vi "CalculateAngleStagetoStave.vi"(0 "Coordinates from images":dbl[][](array[numeric])=[[-618.0000019526123, 132.09984513301268, 23.216226053071207], [-618.0000015711425, 132.10001145381347, 23.216226053071207], [-618.0000001215576, 132.1000061132373, 23.216226053071207], [-606.0002838354981, 132.10000000972167, 23.216226053071207], [-605.9999977332031, 132.10000084895506, 23.216226053071207], [-605.9999913245117, 132.10000268000977, 23.216226053071207], [-337.9510112720312, 132.10002915400878, 23.21612605307121], [-337.9500060230078, 132.10001061458007, 23.216226053071207], [-337.95000091131345, 132.1000039007129, 23.216226053071207], [-325.94987751994137, 132.10000496882813, 23.216226053071207], [-325.9500149253368, 132.10000496882813, 23.216226053071207], [-325.9500006583691, 132.10000573176757, 23.216226053071207], [-43.949846358593746, 132.09996766108887, 23.216226053071207], [-43.950016265209946, 132.09999520320312, 23.216226053071207], [-43.94999185114746, 132.10000382441893, 23.216226053071207], [-31.950448924521478, 132.10000634211914, 23.21612605307121], [-31.94999062679199, 132.10001427668945, 23.216226053071207], [-31.95000397823242, 132.10000313777343, 23.216226053071207], [250.04977136382323, 132.10009530085938, 23.216226053071207], [250.04998895415525, 132.09999756831542, 23.216226053071207], [250.04999795684077, 132.10000405330078, 23.216226053071207], [262.0491744629883, 132.1000239660205, 23.21612605307121], [262.04998653574216, 132.10000451106444, 23.216226053071207], [262.05000721140135, 132.1000140478076, 23.216226053071207]], 1 "Templates path":path=path "C:/Users/Aerotech/Documents/BNL_ThermomechanicalStave/0_Calibration", 2 "Image Array":T1[](array[typedef])=["image_000_-618_132_23", "image_001_-618_132_23", "image_002_-618_132_23", "image_003_-606_132_23", "image_004_-606_132_23", "image_005_-606_132_23", "image_006_-338_132_23", "image_007_-338_132_23", "image_008_-338_132_23", "image_009_-326_132_23", "image_010_-326_132_23", "image_011_-326_132_23", "image_012_-44_132_23", "image_013_-44_132_23", "image_014_-44_132_23", "image_015_-32_132_23", "image_016_-32_132_23", "image_017_-32_132_23", "image_018_250_132_23", "image_019_250_132_23", "image_020_250_132_23", "image_021_262_132_23", "image_022_262_132_23", "image_023_262_132_23"], 3 "Pixel resolution":dbl=1.529578681813674 format="%#_13g", 5 "Number of images each":i32=3, 7 "Number of pins":i32=4) -> (4 "Angle":dbl=0.0006856978788182783, 6 "Locations pins":dbl[][](array[numeric])=[[-609.3870429531735, -329.18563865969537, -35.10730846902823, 259.01426916444484], [134.0388179973662, 135.08170067352683, 134.8703908188264, 134.78325815098862]], 8 "Each point on located edges":T3(graph)=[{"Top averages"=[-601.3926714238871, -617.3814144824598, nan, -323.4827145583182, -334.88856276107254, nan, -29.406789160441058, -40.80782777761541, nan, 264.732596858135, 253.29594147075468, nan, -609.3870429531735, -609.3870429531735, -609.3870429531735, -329.18563865969537, -329.18563865969537, -329.18563865969537, -35.10730846902823, -35.10730846902823, -35.10730846902823, 259.01426916444484, 259.01426916444484, 259.01426916444484], "Best Linear Fit"=[134.0388179973662, 134.0388179973662, 134.0388179973662, 135.08170067352683, 135.08170067352683, 135.08170067352683, 134.8703908188264, 134.8703908188264, 134.8703908188264, 134.78325815098862, 134.78325815098862, 134.78325815098862, 134.09820366135074, 133.97943233338168, nan, 135.73823170843656, 134.4251696386171, nan, 135.57292450870293, 134.16785712894986, nan, 135.40219923996895, 134.16431706200828, nan]}, {"Top averages"=[-700.0, -300.0, 100.0, 500.0, 700.0], "Best Linear Fit"=[134.3360645312021, 134.61034372571643, 134.88462292023075, 135.15890211474508, 135.29604171200225]}])   [LabVIEW 2016]
uses:
  <vilib>/Analysis/6fits.llb/Curve Fitting Criteria.ctl
  <vilib>/vision/Image Controls.llb/IMAQ Image.ctl
  <vilib>/Analysis/NI_AALPro.lvlib
panel:
  in  "Testing?":bool=TRUE
  out "Point for each edge- units":dbl[][][](array[numeric])=[[[-616.6853013924161, 133.98498133920288, 23.19072534]], [[-602.0918631529712, 134.0873275784507, 23.19072534]], [[-616.6844686564219, 133.98510562595666, 23.19072534]], [[-602.0873483929206, 134.10375101417594, 23.19072534]], [[-616.6848465163853, 133.9845728817171, 23.19072534]], [[-602.0884296079262, 134.087169544694, 23.19072534]], [[-334.3899800940794, 135.67998739590436, 23.19072534]], [[-323.9779865268114, 134.48344180918818, 23.19072534]], [[-334.3927140881534, 135.68204709551367, 23.19072534]], [[-323.98295164227596, 134.48329915078338, 23.19072534]], [[-334.3923216504359, 135.6810484407434, 23.19072534]], [[-323.97787795641597, 134.480380149028, 23.19072534]], [[-40.3112304344497, 135.51048660072627, 23.19072534]], [[-29.903300498442807, 134.22953193062764, 23.19082534]], [[-40.31259391421408, 135.5137627222535, 23.19072534]], [[-29.90268539871824, 134.2294673759651, 23.19072534]], [[-40.309615844169045, 135.51088795666246, 23.19072534]], [[-29.90442472417554, 134.2282083267235, 23.19072534]], [[253.79560124818477, 135.34840869395944, 23.19082534]], [[264.2326481830148, 134.22077460141287, 23.19082534]], [[253.79296388701863, 135.34828494250544, 23.19072534]], [[264.2354027367716, 134.217503625029, 23.19072534]], [[253.79395739751806, 135.34811629532663, 23.19072534]], [[264.23504153416127, 134.2164607476983, 23.19072534]]]
  in  "Coordinate file for image capture":path=path "C:/Users/Aerotech/cernbox/BNL/Stave Assembly Records/2017-04-07/staveCalib/staveCoordinatesSystemCaptured.csv"
  out "Filenames Array":string[](array[string])=["image_000_-618_132_23.png", "image_001_-618_132_23.png", "image_002_-618_132_23.png", "image_003_-606_132_23.png", "image_004_-606_132_23.png", "image_005_-606_132_23.png", "image_006_-338_132_23.png", "image_007_-338_132_23.png", "image_008_-338_132_23.png", "image_009_-326_132_23.png", "image_010_-326_132_23.png", "image_011_-326_132_23.png", "image_012_-44_132_23.png", "image_013_-44_132_23.png", "image_014_-44_132_23.png", "image_015_-32_132_23.png", "image_016_-32_132_23.png", "image_017_-32_132_23.png", "image_018_250_132_23.png", "image_019_250_132_23.png", "image_020_250_132_23.png", "image_021_262_132_23.png", "image_022_262_132_23.png", "image_023_262_132_23.png"]
  in  "Naming Convention":string="*.png"
  in  "Images Directory":path=path "C:/Users/Aerotech/cernbox/BNL/Stave Assembly Records/2017-04-07/staveCalib"
  out "y errors (mm)":dbl[](array[numeric])=[0.05938566398452695, 0.6565310349097196, 0.7025336898765229, 0.618941088980328]
  out "x errors (mm)":dbl[](array[numeric])=[7.994371529286357, 5.702924101377151, 5.700519308587177, 5.718327693690156]
  out "Residue":dbl=0.10525358201266499
  in  "x values for fit line on plot":dbl[](array[numeric])=[-700.0, -300.0, 100.0, 500.0, 700.0]
  out "Intercept":dbl=134.81605312160218
  in  "method":T2 items=["Least Square", "Least Absolute Residual", "Bisquare"]
  out "Slope":dbl=0.0006856979862858028
  out "Coordinate array for image capture":dbl[][](array[numeric])=[[-618.000367587, 132.100003781, 23.19072534], [-617.999992679, 132.100009503, 23.19072534], [-617.999994586, 132.100002178, 23.19072534], [-606.000466212, 132.10001202, 23.19072534], [-606.000010661, 132.100002941, 23.19072534], [-606.000002574, 132.100001492, 23.19072534], [-337.950002777, 132.100039486, 23.19072534], [-337.949993164, 132.100003857, 23.19072534], [-337.950002166, 132.099999279, 23.19072534], [-325.950148016, 132.100036511, 23.19072534], [-325.950009619, 132.100006069, 23.19072534], [-325.94999314, 132.099999279, 23.19072534], [-43.950092517, 132.099999279, 23.19072534], [-43.950004092, 132.099999279, 23.19072534], [-43.949995929, 132.100005917, 23.19072534], [-31.949232604, 132.09996014, 23.19082534], [-31.949993789, 132.100005001, 23.19072534], [-31.949996841, 132.100002178, 23.19072534], [250.05059477, 132.10003468, 23.19082534], [250.050008299, 132.099999432, 23.19072534], [250.050006239, 132.100006298, 23.19072534], [262.050305181, 132.100005917, 23.19082534], [262.050004125, 132.099996685, 23.19072534], [262.050004965, 132.100004086, 23.19072534]]
  out "Images Array":T1[](array[plugin-control])=["image_000_-618_132_23", "image_001_-618_132_23", "image_002_-618_132_23", "image_003_-606_132_23", "image_004_-606_132_23", "image_005_-606_132_23", "image_006_-338_132_23", "image_007_-338_132_23", "image_008_-338_132_23", "image_009_-326_132_23", "image_010_-326_132_23", "image_011_-326_132_23", "image_012_-44_132_23", "image_013_-44_132_23", "image_014_-44_132_23", "image_015_-32_132_23", "image_016_-32_132_23", "image_017_-32_132_23", "image_018_250_132_23", "image_019_250_132_23", "image_020_250_132_23", "image_021_262_132_23", "image_022_262_132_23", "image_023_262_132_23"]
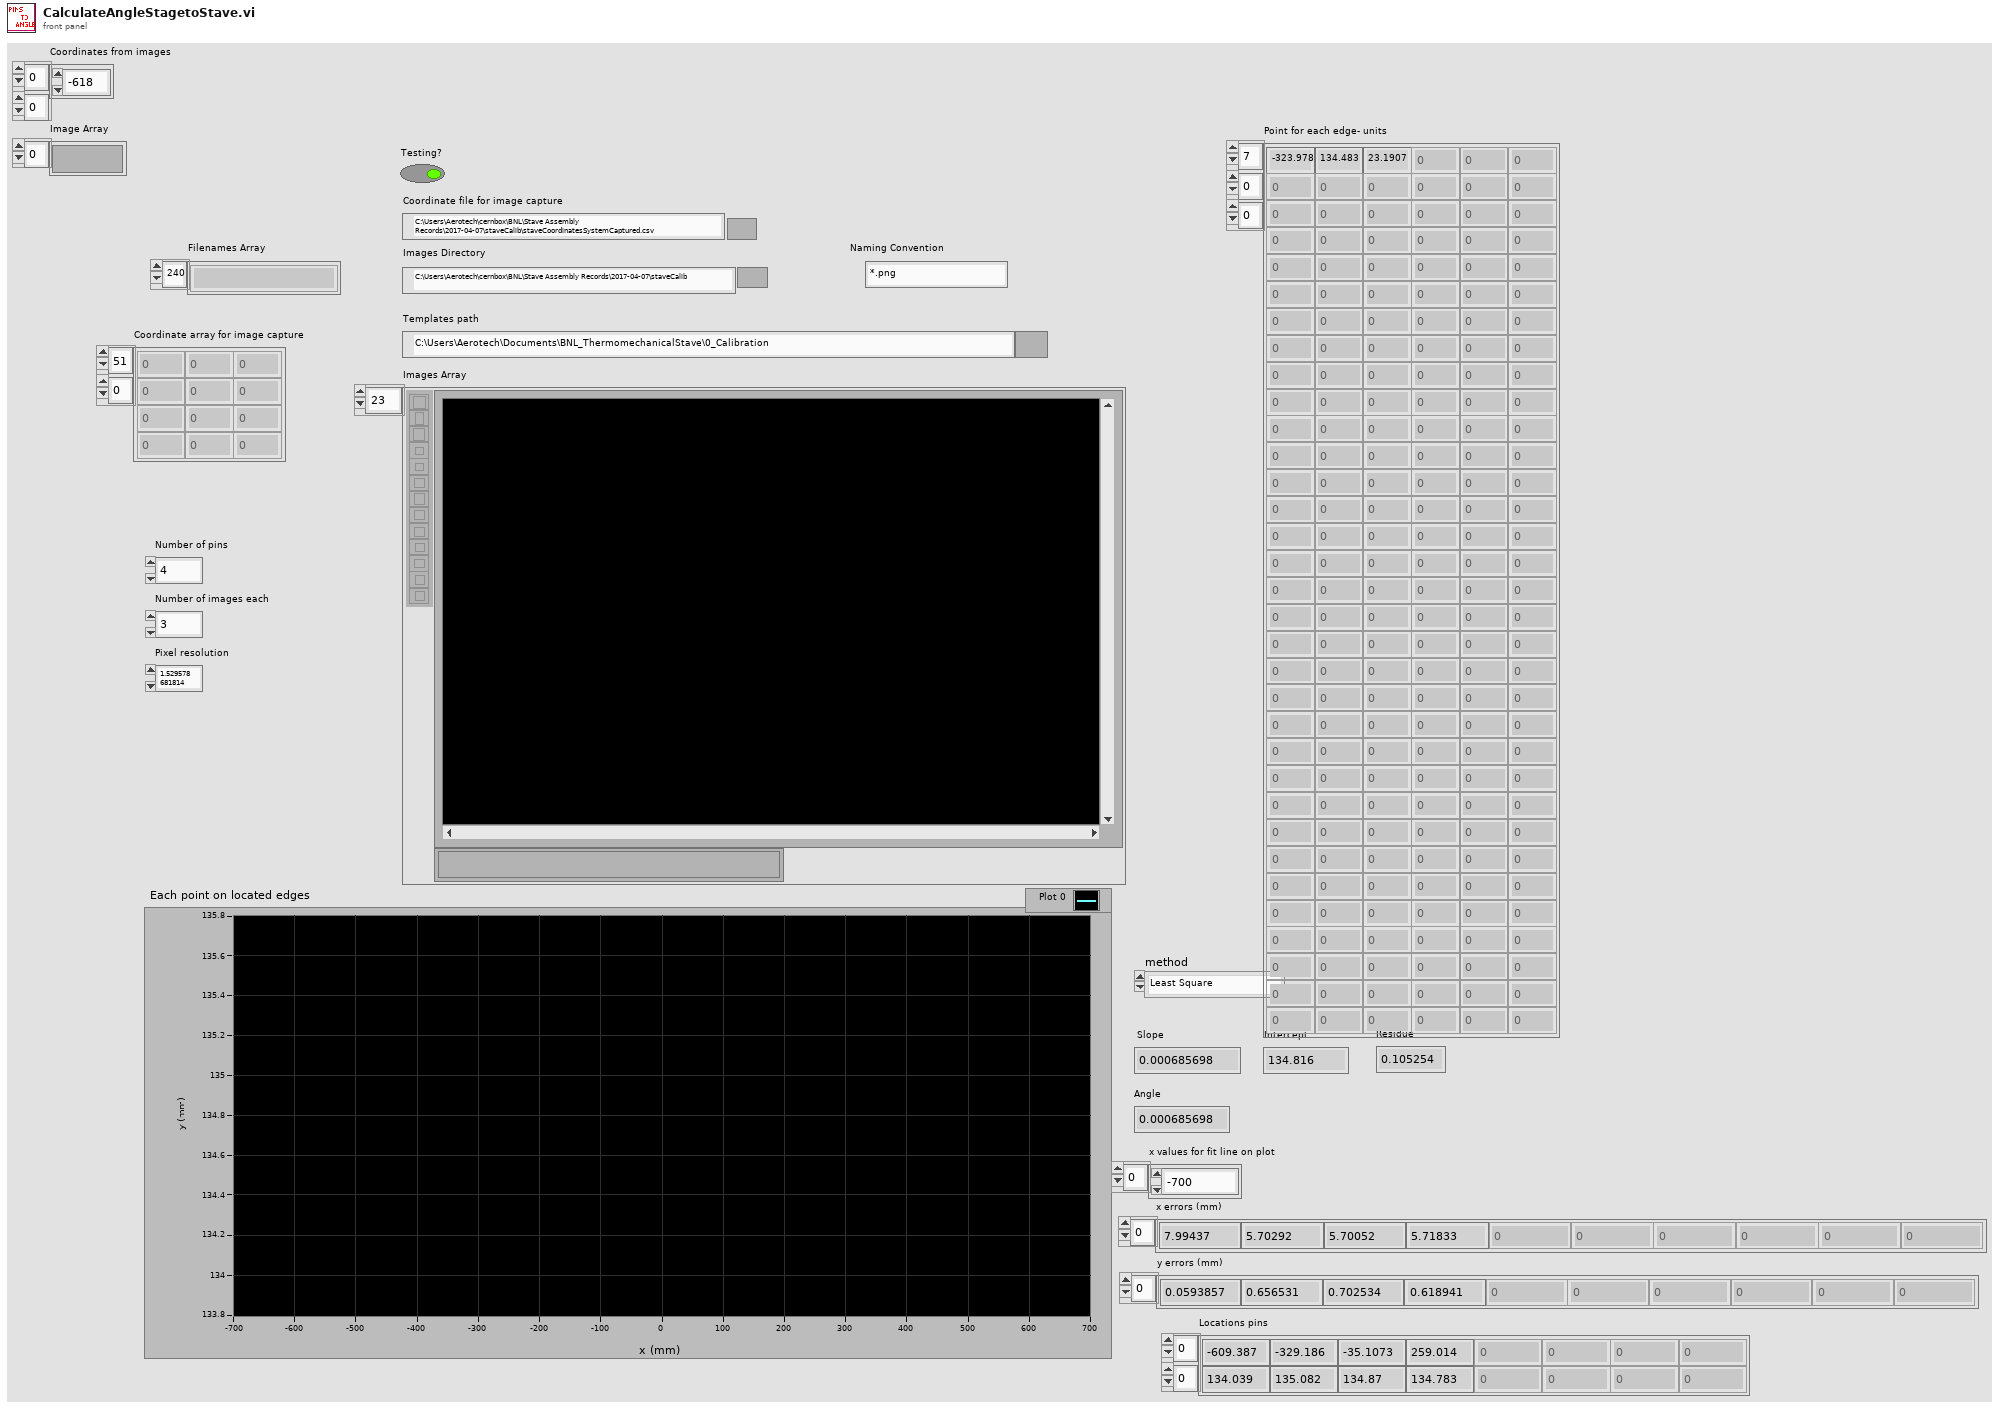
[diagram p1: front panel]
types:
  T1 = typedef "IMAQ Image.ctl" = refnum<image>
  T2 = typedef "NI_AALPro.lvlib/Curve Fitting Criteria.ctl" = u16
  T3 = cluster{"Top averages":dbl[], "Best Linear Fit":dbl[]}[]
  T4 = enum16{"cm", "mm", "pixels [mm/pix]", "pixels [um/pix]"}
  T5 = cluster{"Top Averages":dbl[], "Top Averages":dbl[]}
  T6 = cluster{"x values for fit line on plot":dbl[], "Array":dbl[]}
  T7 = cluster{"x values for fit line on plot":dbl[], "Array":dbl[]}[]
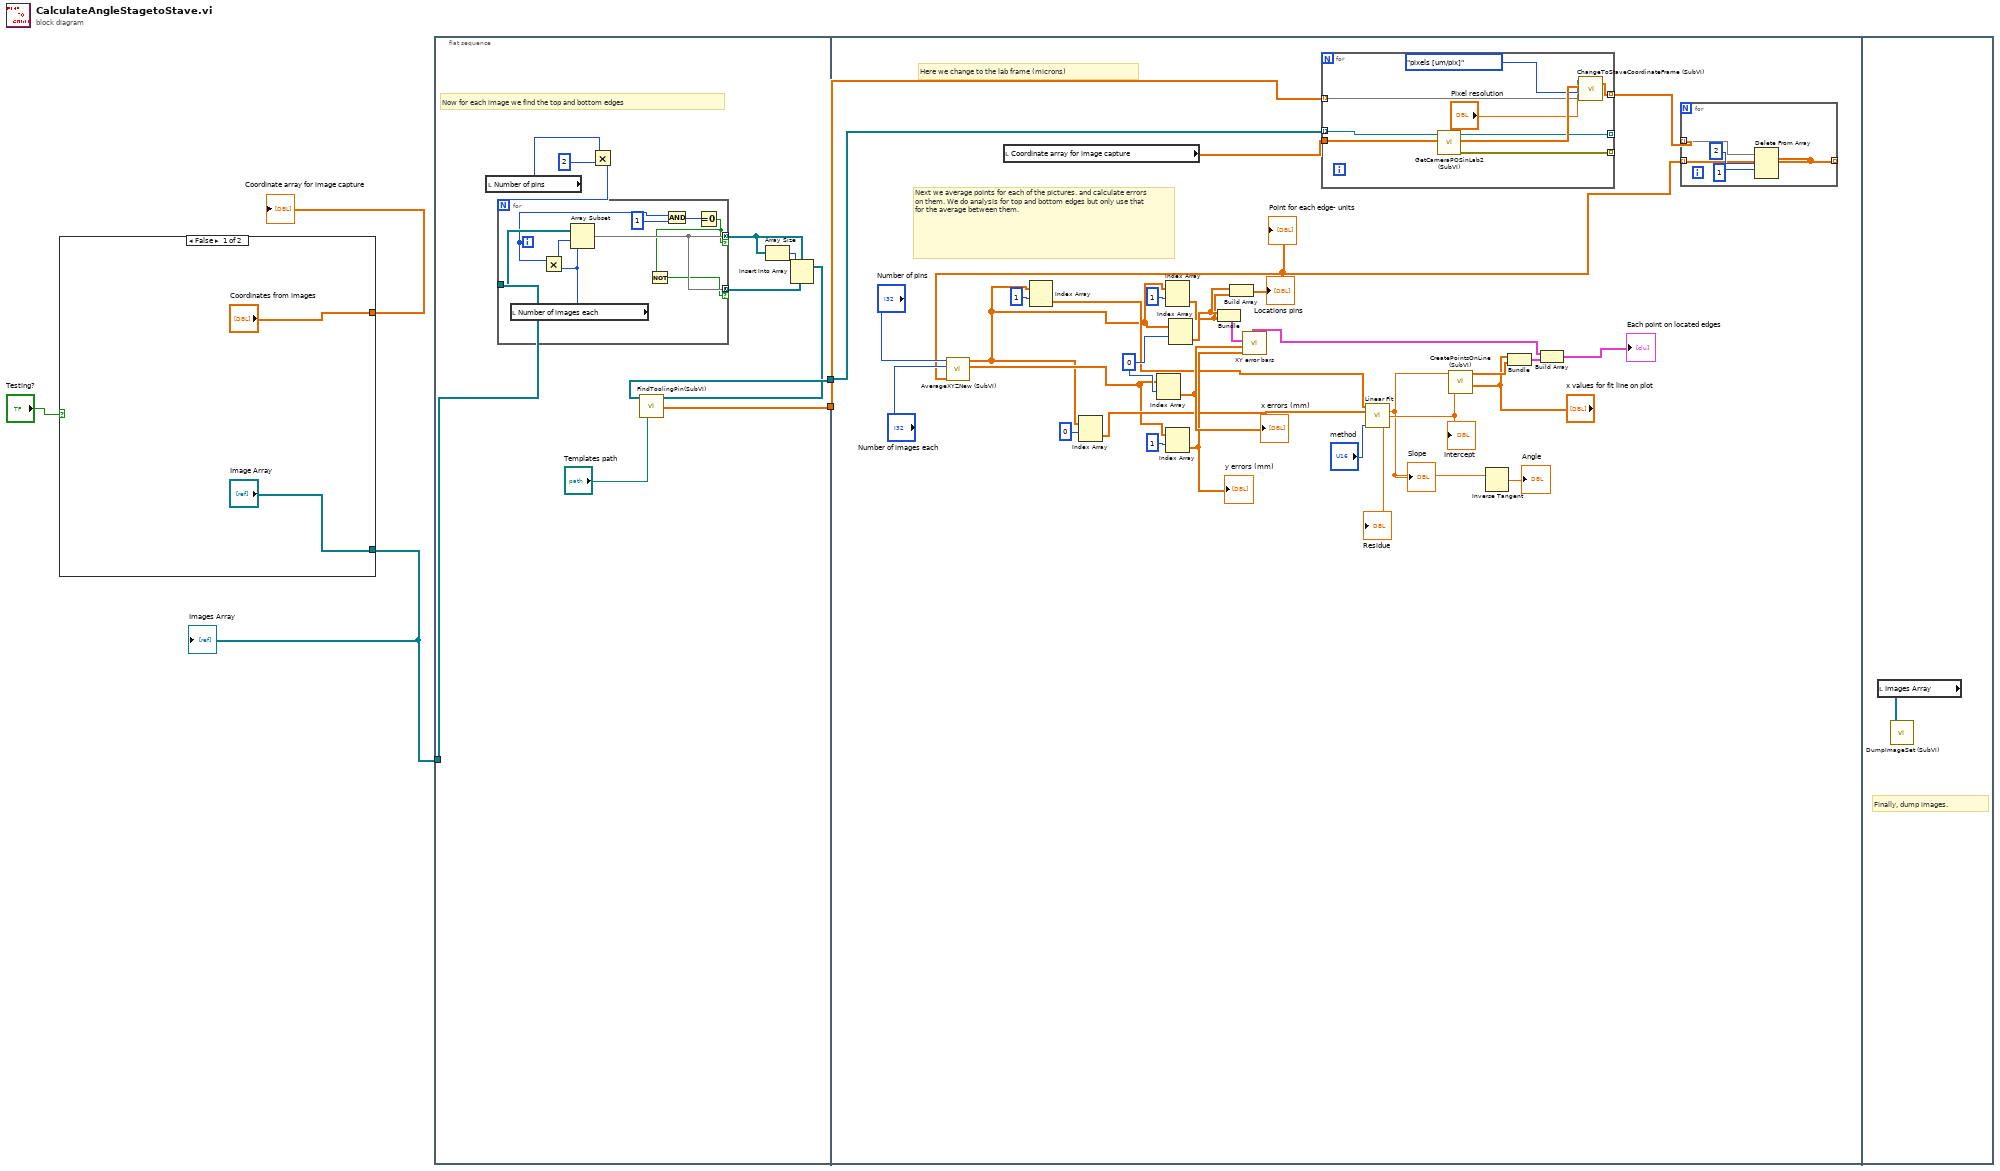
[diagram p0: block diagram]
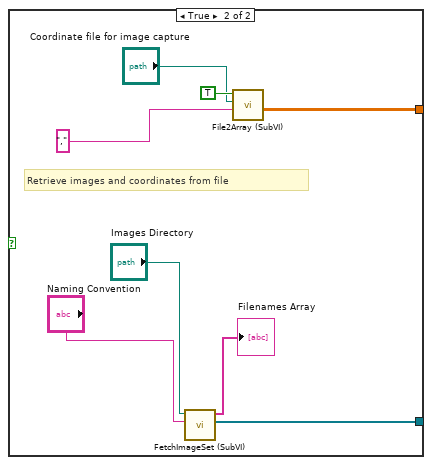
[diagram p2: hidden frame]
diagram:
  n1 = case shown="False" "Testing?" {
    tunnel: ["Coordinates from images" w9] -> w5
    tunnel: ["Image Array" w8] -> w4
    frame False {
    }
    frame True {
      # "Retrieve images and coordinates from file"
      n2 = call "FetchImageSet (SubVI).vi"("Naming Convention"="Naming Convention", "Images Directory"="Images Directory") -> ("Image Array"=w8:T1[], "Filenames Array"=→"Filenames Array":string[])  [unwired: 7 in, 1 out]
      n3 = call "File2Array (SubVI).vi"("File delimiter"=",", "Source array file"="Coordinate file for image capture", "Load array from file?"=TRUE) -> ("Loaded array"=w9:dbl[][])  [unwired: 7 in, 1 out]
    }
  }
  "Images Array" <- w4
  "Coordinate array for image capture" <- w5
  n4 = flat-sequence {
    tunnel: w4 -> [w23]
    tunnel: [w26] -> w3
    tunnel: [w24] -> w2
    tunnel: w3 -> [w67]
    tunnel: w2 -> [w43]
    frame #0 {
      # "Now for each image we find the top and bottom edges"
      n5 = local read "Number of pins"() -> (w18:i32)
      n6 = Multiply(x=w18, y=2) -> (x*y=w16:i32)
      n7 = for {
        N: w16 -> [_]
        tunnel: w23 -> [w35]
        tunnel: [w32] -> w19 mode=concatenating if=w28
        tunnel: [w32] -> w21 mode=concatenating if=w27
        i -> [w31]
        n8 = local read "Number of images each"() -> (w34:i32)
        n9 = Multiply(x=w31, y=w34) -> (x*y=w33:i32)
        n10 = Array Subset(array=w35, index=w33, length=w34) -> (w32:T1[])
        n11 = And(x=w31, y=1) -> (x .and. y?=w29:i32)
        n12 = Equal To 0?(x=w29) -> (x = 0?=w28:bool)
        n13 = Not(x=w28) -> (.not. x?=w27:bool)
      }
      n14 = Array Size(array=w19) -> (size(s)=w20:i32)
      n15 = Insert Into Array(array=w19, index=w20, new element=w21) -> (w22:T1[])
      n16 = call "FindToolingPin(SubVI).vi"("Calibrated Image Array"=w22, "Templates path"="Templates path") -> ("Analyzed Image Array"=w26:T1[], "Center positions"=w24:sgl[][][])  [unwired: 12 in]
    }
    frame #1 {
      w64 = 0 ("index (row)")
      # "Next we average points for each of the pictures. and calculate errors on them. We do analysis for top and bottom edges but only use that for the average between them."
      # "Here we change to the lab frame (microns)"
      n17 = local read "Coordinate array for image capture"() -> (w66:dbl[][])
      n18 = for {
        tunnel: w67 -> [w80] mode=indexing
        tunnel: w66 -> [w79]
        tunnel: [w75] -> _ mode=indexing
        tunnel: [w74] -> w42 mode=indexing
        tunnel: [w73] -> _ mode=indexing
        tunnel: w43 -> [w72] mode=indexing
        n19 = call "GetCameraPOSinLab2 (SubVI).vi"("Loaded array"=w79, "Refnum in"=w80) -> ("error out"=w75:errorcluster, "Image coordinates in lab frame"=w78:dbl[], "Refnum out"=w73:T1)  [unwired: 7 in]
        n20 = call "ChangeToStaveCoordinateFrame (SubVI).vi"("Loaded array (image frame)"=w72, "Image Origin in XYZ Stage Coords [mm]"=w78, "Units"=T4."pixels [um/pix]", "Pixel resolution"="Pixel resolution") -> ("Array (stage frame, mm)"=w74:dbl[][])  [unwired: 2 in]
      }
      n21 = for {
        tunnel: w42 -> [w71] mode=indexing
        tunnel: [w68] -> _ mode=indexing
        tunnel: [w68] -> w41 mode=indexing
        n22 = Delete From Array(array=w71, length=2, index (row)=1) -> (array with subset deleted=w68:dbl[][])  [unwired: 1 in, 1 out]
      }
      "Point for each edge- units" <- w41
      n23 = call "AverageXYZNew (SubVI).vi"("array"=w41, "Number of images each"="Number of images each", "Number of pins"="Number of pins") -> ("Top uncertainty"=w45:dbl[][], "Top Averages"=w44:dbl[][])  [unwired: 7 in]
      n24 = Index Array(array=w44, index (row)=1) -> (element=w58:dbl[])  [unwired: 1 in]
      n25 = Index Array(array=w44, index (row)=0) -> (element=w57:dbl[])  [unwired: 1 in]
      n26 = Index Array(array=w45, index (row)=w64) -> (element=w62:dbl[])  [unwired: 1 in]
      "x errors (mm)" <- w62
      n27 = Index Array(array=w44, index (row)=1) -> (element=w39:dbl[])  [unwired: 1 in]
      n28 = Index Array(array=w45, index (row)=1) -> (element=w61:dbl[])  [unwired: 1 in]
      "y errors (mm)" <- w61
      n29 = Index Array(array=w44, index (row)=w64) -> (element=w40:dbl[])  [unwired: 1 in]
      n30 = Bundle("Top Averages"=w40, "Top Averages"=w39) -> (w63:T5)  [unwired: 1 in]
      n31 = Build Array(w40, w39) -> (→"Locations pins":dbl[][])
      n32 = call "XY error bars.vi"("XY plot"=w63, "Xerror"=w62, "Yerror"=w61) -> ("X+Y error bars"=w56:cluster{dbl[], dbl[]})  [unwired: 5 in, 2 out]
      n33 = call <vilib>:"Linear Fit.vi"("Y"=w58, "X"=w57, "method"="method") -> ("slope"=w37:dbl, "intercept"=w52:dbl, "residue"=→"Residue":dbl)  [unwired: 8 in, 2 out]
      "Slope" <- w37
      "Intercept" <- w52
      n34 = call "CreatePointsOnLine (SubVI).vi"("x values for fit line on plot"="x values for fit line on plot", "intercept"=w52, "slope"=w37) -> ("Array"=w51:dbl[])  [unwired: 8 in]
      n35 = Inverse Tangent(1:w37) -> (0:→"Angle":dbl)
      n36 = Bundle("x values for fit line on plot"="x values for fit line on plot", "Array"=w51) -> (w50:T6)  [unwired: 1 in]
      n37 = Build Array(w56, w50) -> (→"Each point on located edges":T7)
    }
    frame #2 {
      # "Finally, dump images."
      n38 = local read "Images Array"() -> (w81:T1[])
      n39 = call "DumpImageSet (SubVI).vi"("Calibrated Image Array"=w81) -> ()  [unwired: 7 in, 1 out]
    }
  }
